vi "Get Properties and Commands Used.vi"(8 "error in (no error)":errorcluster, 10 "relays":i32[](array[numeric]), 11 "SLSC Switch in":refnum<class "SLSC Switch.lvclass">) -> (0 "error out":errorcluster, 1 "commands":refnum<k21>[](array[refnum]), 2 "properties":refnum<k21>[](array[refnum]), 3 "SLSC Switch out":refnum<class "SLSC Switch.lvclass">)   [LabVIEW 2015, in "SLSC Switch.lvclass"]
uses:
  SLSC Switch.lvclass
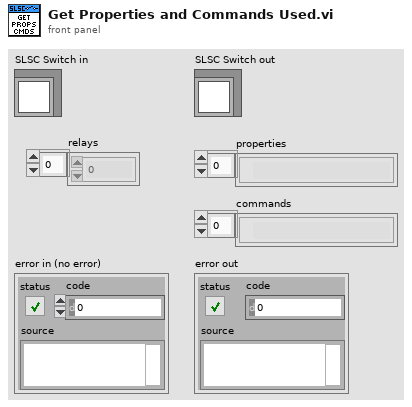
[diagram p1: front panel]
types:
  T1 = typedef "SLSC Switch.lvclass/SLSC Relay Info.ctl" = cluster{"property":refnum<k21>, "command":refnum<k21>}
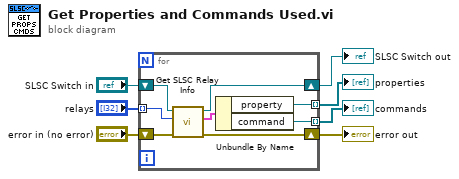
[diagram p0: block diagram]
diagram:
  n1 = for {
    tunnel: "relays" -> [w14] mode=indexing
    shift-right: [w13] -> w3
    shift-left: "SLSC Switch in" -> [w15]
    tunnel: [w11] -> w2 mode=indexing
    shift-right: [w10] -> w4
    shift-left: "error in (no error)" -> [w9]
    tunnel: [w8] -> w1 mode=indexing
    n2 = call "Get SLSC Relay Info.vi"("error in (no error)"=w9, "relay index"=w14, "SLSC Switch in"=w15) -> ("error out"=w10:errorcluster, "SLSC Switch Info"=w12:T1, "SLSC Switch out"=w13:refnum<class "SLSC Switch.lvclass">)  [unwired: 6 in]
    n3 = Unbundle By Name(w12) -> ("property"=w11:refnum<k21>, "command"=w8:refnum<k21>)
  }
  "error out" <- w4
  "commands" <- w1
  "SLSC Switch out" <- w3
  "properties" <- w2
